vi "Make VI Param(Read Profile Rsp).vi"(1 "pRsp":T1) -> (0 "Read Profile Rsp":T2)   [LabVIEW 2014, in "Keyence LJ-V7000.lvlib"]
uses:
  Keyence LJ-V7000.lvlib
  Public/Clusters/Read Profile Rsp.ctl
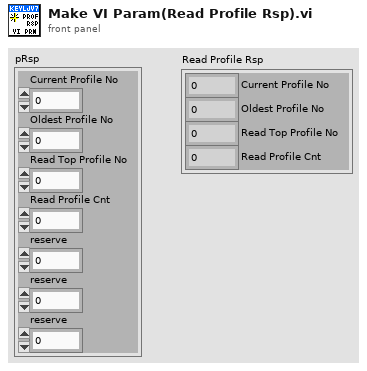
[diagram p1: front panel]
types:
  T1 = cluster{"Current Profile No":u32, "Oldest Profile No":u32, "Read Top Profile No":u32, "Read Profile Cnt":u8, "reserve":u8, "reserve":u8, "reserve":u8}
  T2 = typedef "Keyence LJ-V7000.lvlib/Read Profile Rsp.ctl" = cluster{"Current Profile No":u32, "Oldest Profile No":u32, "Read Top Profile No":u32, "Read Profile Cnt":u8}
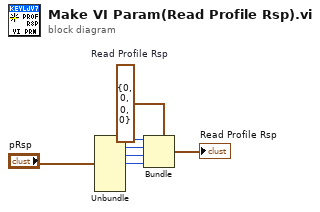
[diagram p0: block diagram]
diagram:
  w3 = T2 {"Current Profile No"=0, "Oldest Profile No"=0, "Read Top Profile No"=0, "Read Profile Cnt"=0}  # Read Profile Rsp
  n1 = Unbundle("pRsp") -> ("Current Profile No"=w7:u32, "Oldest Profile No"=w6:u32, "Read Top Profile No"=w5:u32, "Read Profile Cnt"=w4:u8)  [unwired: 3 out]
  n2 = Bundle(cluster=w3, "Current Profile No"=w7, "Oldest Profile No"=w6, "Read Top Profile No"=w5, "Read Profile Cnt"=w4) -> (→"Read Profile Rsp":T2)
